vi "DFD FXP NStage MRate Quantization.vi"(5 "scale by power of 2? (F)":bool, 6 "gain settings":T1={"gain processing"=1, "gain word length"=16} {"gain processing" items=["On Target", "On Host"]}, 7 "scale type":T4=enum."Time Domain 1-Norm", 8 "error in (no error)":errorcluster, 10 "coefficients word lengths":i16[](array[numeric]), 11 "multirate filters in":T2[](array[typedef]) {"mMRate_SumWl" min=1 max=32 step=1; "mMRate_InputIwl" min=1 max=32 step=1; "mMRate_GainWl" min=1 max=32 step=1; "mMRate_OutputWl" min=1 max=32 step=1; "mMRate_InputWl" min=1 max=32 step=1; "mMRate_CoefWl" min=1 max=32 step=1; "mMRate_Mode" items=["Default"=-1, "No Rate Change"=0, "Interpolation"=1, "Decimation"=2, "Interpolated"=3, "Rational"=4]}) -> (0 "error out":errorcluster, 2 "postprocessing gain":dbl, 3 "multirate filters out":T2[](array[typedef]) {"mMRate_SumWl" min=1 max=32 step=1; "mMRate_InputIwl" min=1 max=32 step=1; "mMRate_GainWl" min=1 max=32 step=1; "mMRate_OutputWl" min=1 max=32 step=1; "mMRate_InputWl" min=1 max=32 step=1; "mMRate_CoefWl" min=1 max=32 step=1; "mMRate_Mode" items=["Default"=-1, "No Rate Change"=0, "Interpolation"=1, "Decimation"=2, "Interpolated"=3, "Rational"=4]})   [LabVIEW 2017, in "NI_DigFilterLicensed.lvlib"]
doc: "Quantizes the coefficients of a floating-point multistage multirate filter and generates a fixed-point multistage multirate filter. This VI has the same internal settings as the DFD FXP MRate Quantization VI."
uses:
  <vilib>/addons/Digital Filter Design/NI_DigFilterLicensed.lvlib
  <vilib>/addons/Digital Filter Design/_Objects.llb/DFD Coef Norm Type.ctl
  <vilib>/addons/Digital Filter Design/_Objects.llb/DFD Multirate Filter Obj.ctl
  <vilib>/addons/Digital Filter Design/_Objects.llb/DFD Multirate Mode.ctl
  <vilib>/addons/Digital Filter Design/_Objects.llb/DFD Round-off Mode.ctl
  <vilib>/addons/Digital Filter Design/_Objects.llb/DFD FXP MRate Multiply Mode.ctl
  <vilib>/addons/Digital Filter Design/NI_DigFilter_FXP.lvlib
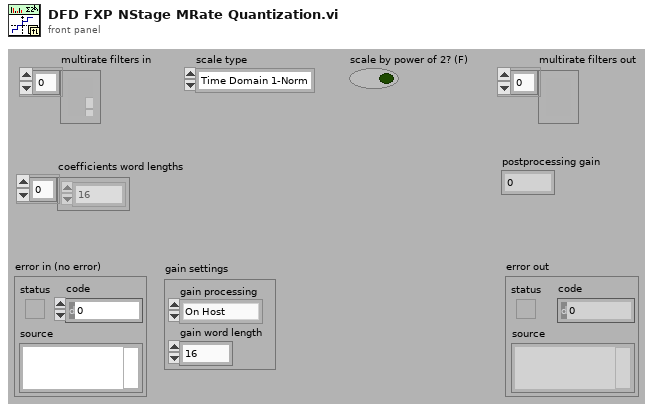
[diagram p1: front panel]
types:
  T1 = cluster{"gain processing":u16, "gain word length":i16}
  T2 = typedef "NI_DigFilterLicensed.lvlib/DFD Multirate Filter Obj.ctl" = cluster{"mMRate_Structure":enum16{"CIC", "FIR", "IIR", "Lattice"}, "mMRate_Mode":T3, "mMRate_Factor":i32, "mMRate_FIRParams":cluster{"mMRate_FIR_H":dbl[], "mMRate_FIR_IsNyquist?":bool, "mMRate_FIR_IsSymmetric?":bool}, "mMRate_CICParams":cluster{"mMRate_CIC_#Stage":i32, "mMRate_CIC_Lag":i32, "mMRate_CIC_Type":enum16{"Lowpass", "Highpass"}}, "mMRate_Order":i32, "mMRate_Version":string, "mMRate_Comments":string, "mMRate_RationalFactor":cluster{"mMRate_L":i32, "mMRate_M":i32}, "mMRate_Fs":dbl, "mMRate_Quantized?":bool, "mMRate_QFilterGain":dbl, "mMRate_CoefWl":i16, "mMRate_Scaling":cluster{"mMRate_ScaleByPowerOf2?":bool, "mMRate_ScaleType":T4}, "mMRate_InputWl":i16, "mMRate_OutputWl":i16, "mMRate_OutputMode":T5, "mMRate_MultMode":T6, "mMRate_BitPruning":bool, "mMRate_GainWl":i16, "mMRate_OutputFwl":i16, "mMRate_SumIwl":i16, "mMRate_InputIwl ":i16, "mMRate_SumWl":i16, "mMRate_CoefIwl":i16}
  T3 = typedef "NI_DigFilterLicensed.lvlib/DFD Multirate Mode.ctl" = i16
  T4 = typedef "NI_DigFilterLicensed.lvlib/DFD Coef Norm Type.ctl" = enum16{"No Norm", "Time Domain 1-Norm", "Time Domain 2-Norm", "Time Domain Inf-Norm"}
  T5 = typedef "NI_DigFilterLicensed.lvlib/DFD Round-off Mode.ctl" = enum16{"Nearest", "Truncation"}
  T6 = typedef "NI_DigFilterLicensed.lvlib/DFD FXP MRate Multiply Mode.ctl" = enum16{"Truncated", "Full"}
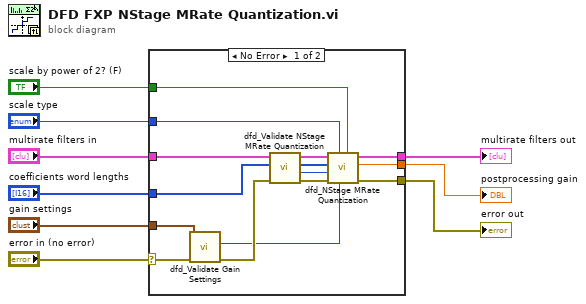
[diagram p0: block diagram]
diagram:
  n1 = case shown="No Error" "error in (no error)" {
    selector: "error in (no error)" -> [w10 w25]
    tunnel: "multirate filters in" -> [w24 _]
    tunnel: "gain settings" -> [w22 _]
    tunnel: "coefficients word lengths" -> [w21 _]
    tunnel: "scale type" -> [w16 _]
    tunnel: "scale by power of 2? (F)" -> [w15 _]
    tunnel: [w13 _] -> w4
    tunnel: [w12 _] -> w3
    tunnel: [w11 w25] -> w2
    frame No Error {
      n2 = call <vilib>:"dfd_Validate Gain Settings.vi"("error in (no error)"=w10, "gain setting"=w22) -> ("error out"=w23:errorcluster, "gain wl"=w14:i16)  [unwired: 8 out]
      n3 = call <vilib>:"dfd_Validate NStage MRate Quantization.vi"("error in (no error)"=w23, "coef wl"=w21, "multirate filters in"=w24) -> ("error out"=w20:errorcluster, "last FIR idx"=w17:i32, "dup coef wl"=w19:i16[], "dup multirate filters in"=w18:T2[])  [unwired: 5 out]
      n4 = call <vilib>:"dfd_NStage MRate Quantization.vi"("scale by Power of 2?"=w15, "gain wl"=w14, "scale type"=w16, "error in (no error)"=w20, "last FIR idx"=w17, "coef wl"=w19, "multirate filters in"=w18) -> ("error out"=w11:errorcluster, "scaled gain"=w12:dbl, "multirate filters out"=w13:T2[])  [unwired: 2 out]
    }
    frame Error {
    }
  }
  "error out" <- w2
  "postprocessing gain" <- w3
  "multirate filters out" <- w4
